vi "Scratch.vi"() -> ()   [LabVIEW 2012]
panel:
  out "path":path
  out "result string":string
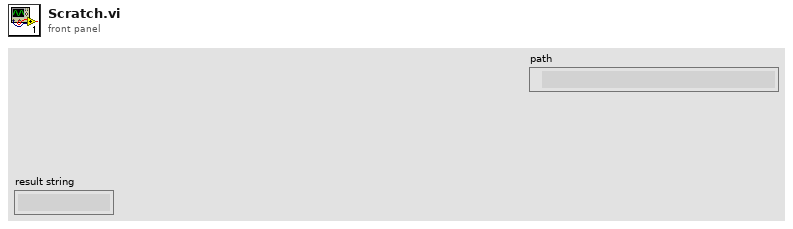
[diagram p1: front panel]
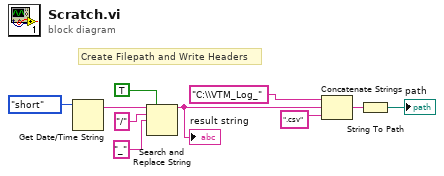
[diagram p0: block diagram]
diagram:
  # "Create Filepath and Write Headers"
  n1 = Get Date/Time String(date format (0)=enum16{"short", "long", "abbreviated"}."short") -> (date string=w9:string)  [unwired: 2 in, 1 out]
  n2 = Search and Replace String(replace all?=TRUE ("replace all? (F)"), input string=w9, search string="/", replace string="_" ("replace string (\"\")")) -> (result string=w5:string)  [unwired: 4 in, 3 out]
  "result string" <- w5
  n3 = Concatenate Strings("C:\\VTM_Log_", w5, ".csv" ("string")) -> (w3:string)
  n4 = String To Path(string=w3) -> (path=→"path":path)
